vi "Exercise 3-6 - Temperature Converter.vi"() -> ()   [LabVIEW 2014]
panel:
  in  "?":bool
  in  "Option":T1(ring)
  out "Output Value":dbl
  out "Input Value":dbl
  in  "Input":dbl(slide) min=-460.0 max=460.0 step=1.0 scale=-273.0..212.0
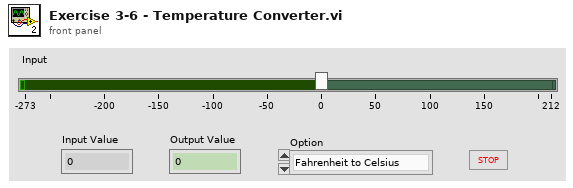
[diagram p1: front panel]
types:
  T1 = enum8{"Fahrenheit to Celsius", "Celsius to Fahrenheit", "Fahrenheit to Kelvin", "Celsius to Kelvin"}
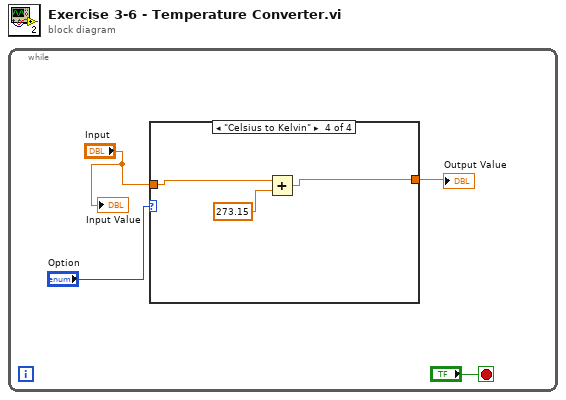
[diagram p0: block diagram]
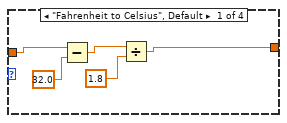
[diagram p2: hidden frame]
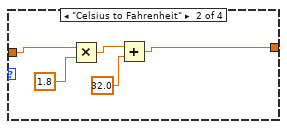
[diagram p3: hidden frame]
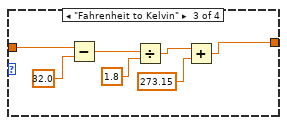
[diagram p4: hidden frame]
diagram:
  n1 = while {
    stop <- "?" stop-if-true
    n2 = case shown="\"Celsius to Kelvin\"" "Option" {
      tunnel: "Input" -> [w9 w13 w19 w23]
      tunnel: [w5 w10 w15 w22] -> w1
      frame "Fahrenheit to Celsius", Default {
        n3 = Subtract(x=w9, y=32.0 ("x-y")) -> (x-y=w6:dbl)
        n4 = Divide(x=w6, y=1.8) -> (x/y=w5:dbl)
      }
      frame "Celsius to Fahrenheit" {
        n5 = Multiply(x=w13, y=1.8) -> (x*y=w12:dbl)
        n6 = Add(x=w12, y=32.0 ("x+y")) -> (x+y=w10:dbl)
      }
      frame "Fahrenheit to Kelvin" {
        n7 = Subtract(x=w19, y=32.0) -> (x-y=w18:dbl)
        n8 = Divide(x=w18, y=1.8) -> (x/y=w17:dbl)
        n9 = Add(x=w17, y=273.15) -> (x+y=w15:dbl)
      }
      frame "Celsius to Kelvin" {
        n10 = Add(x=w23, y=273.15) -> (x+y=w22:dbl)
      }
    }
    "Output Value" <- w1
    "Input Value" <- "Input"
  }
